vi "Write Data.vi"(8 "error in (no error)":errorcluster, 9 "Publication Time":timestamp, 10 "Value":variant, 11 "TerminalReferenceBinding In":refnum<class "TerminalReferenceBinding.lvclass">) -> (0 "error out":errorcluster, 3 "TerminalReferenceBinding Out":refnum<class "TerminalReferenceBinding.lvclass">)   [LabVIEW 2015, in "Transport.lvlib" / "TerminalReferenceBinding.lvclass"]
doc: "<License>\nCopyright © 2017 Composed Systems, LLC | All rights reserved\nwww.composed.io\n\nAuthor: Ethan Stern <ethan.stern@composed.io>\n\nThis software is provided \"AS IS\" WITHOUT WARRANTIES, either express or implied, AND IS FOR EDUCATIONAL PURPOSES ONLY.\n</License>"
uses:
  TerminalReferenceBinding.lvclass
  TerminalReferenceBinding.lvclass/TerminalReferenceBinding.ctl
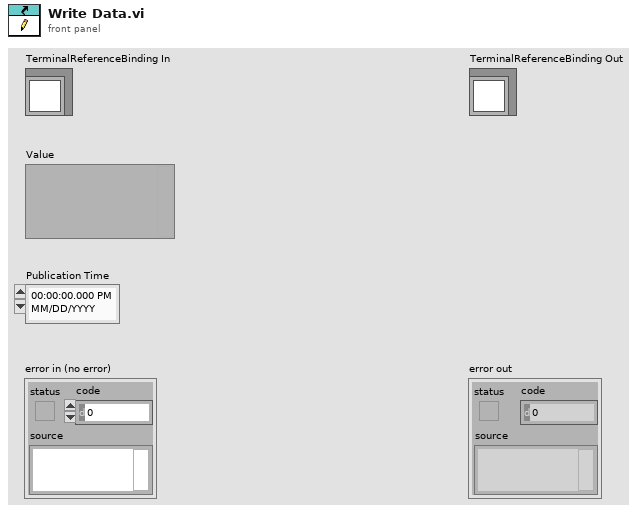
[diagram p1: front panel]
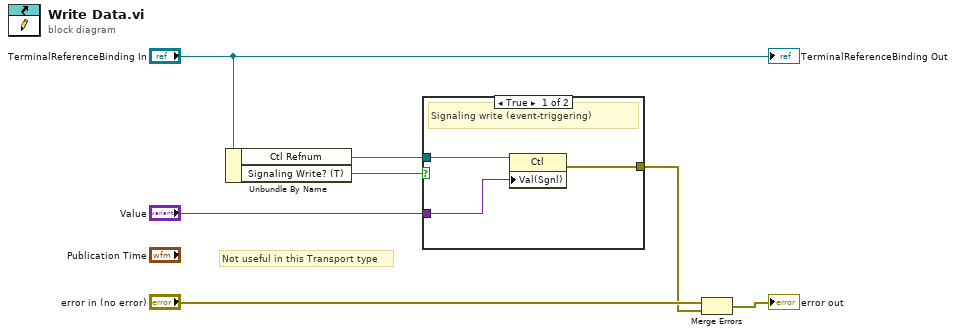
[diagram p0: block diagram]
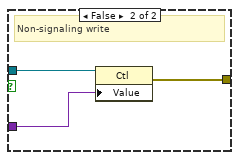
[diagram p2: hidden frame]
diagram:
  # "Not useful in this Transport type"
  n1 = Unbundle By Name("TerminalReferenceBinding In") -> ("Ctl Refnum"=w5:refnum<vi>, "Signaling Write? (T)"=w1:bool)
  n2 = case shown="True" w1 {
    tunnel: w5 -> [w10 w13]
    tunnel: [w9 w12] -> w3
    tunnel: "Value" -> [w8 w11]
    frame True {
      # "Signaling write (event-triggering)"
      n3 = property class="Ctl"(reference=w10, "Val(Sgnl)"=w8) -> (error out=w9:errorcluster)  [unwired: 1 in, 1 out]
    }
    frame False {
      # "Non-signaling write"
      n4 = property class="Ctl"(reference=w13, "Value"=w11) -> (error out=w12:errorcluster)  [unwired: 1 in, 1 out]
    }
  }
  n5 = Merge Errors("error in (no error)", w3) -> (→"error out":errorcluster)
  "TerminalReferenceBinding Out" <- "TerminalReferenceBinding In"
